vi "RSZVB Print.vi"(8 "error in (no error)":errorcluster {"code" format="%.0x"}, 10 "Printer Name":string, 11 "VISA session":refnum<visa-resource-name>) -> (0 "error out":errorcluster {"code" format="%.0x"}, 3 "dup VISA session":refnum<visa-resource-name>)   [LabVIEW 2011]
doc: "This VI prints the active setup on selected printer.\n\nNote(s):\n\nUse Standard Windows Print dialog box to, specify the range of pages to be printed, the number of copies, the destination printer, and other printer setup options.\n\nRemote-control command(s):\nHCOPy:DESTination <string>\nHCOPy[:IMMediate]"
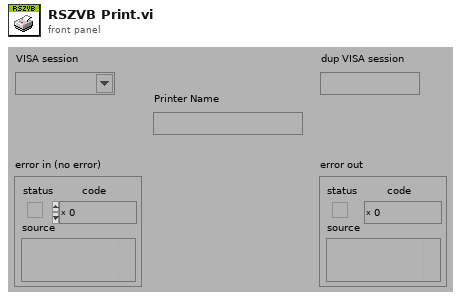
[diagram p1: front panel]
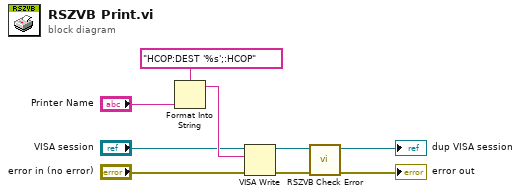
[diagram p0: block diagram]
diagram:
  n1 = Format Into String(format string="HCOP:DEST '%s';:HCOP", "Printer Name") -> (resulting string=w6:string)  [unwired: 2 in, 1 out]
  n2 = VISA Write(VISA resource name="VISA session", write buffer=w6, error in (no error)="error in (no error)") -> (VISA resource name out=w9:refnum<visa-resource-name>, error out=w8:errorcluster)  [unwired: 1 out]
  n3 = call "RSZVB Check Error.vi"("error in (no error)"=w8, "VISA session"=w9) -> ("error out"=→"error out":errorcluster, "dup VISA session"=→"dup VISA session":refnum<visa-resource-name>)  [unwired: 8 in]
